vi "pass_2d_to_DLL.vi"() -> ()   [LabVIEW 2015]
uses:
  C:/Users/MAHA/Desktop/merjeeeee/bin/Debug/merjeeeee.dll
panel:
  out "return type":i32
  in  "Array 2":i32[][](array[numeric])
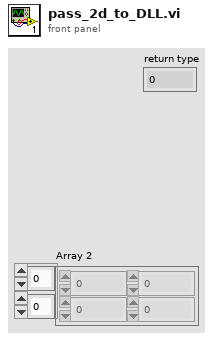
[diagram p1: front panel]
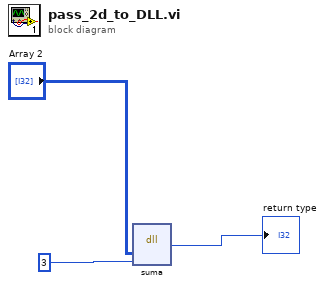
[diagram p0: block diagram]
diagram:
  n1 = dll-call lib="C:/Users/MAHA/Desktop/merjeeeee/bin/Debug/merjeeeee.dll" fn="suma"("n"="Array 2", "m"=3) -> ("return type"=→"return type":i32)  [unwired: 5 in, 2 out]
